vi "Taskbar Setup.vi"(4 "error in (no error)":errorcluster, 5 "DEV Icon Path (empty)":path, 6 "Tooltip Text (\"\")":string, 7 "Window Name (\"\")":string) -> (0 "error out":errorcluster, 1 "hIcon":i32, 2 "hWnd":T2, 3 "siwutil32":T1)   [LabVIEW 2011]
uses:
  SI.LIB/WIN32/WinUSER/Windows/hWnd.ctl
  SI.LIB/WIN32/SIWUTIL32/siwutil32.ctl
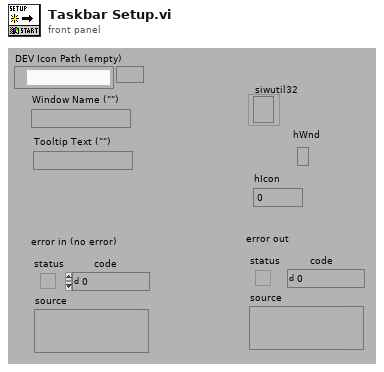
[diagram p1: front panel]
types:
  T1 = typedef "siwutil32.ctl" = refnum<k7>
  T2 = typedef "hWnd.ctl" = refnum<k1>
  T3 = enum32{"invalid app kind", "Development System", "Run Time System", "Student Edition", "Embedded LabVIEW", "Evaluation", "Custom"}
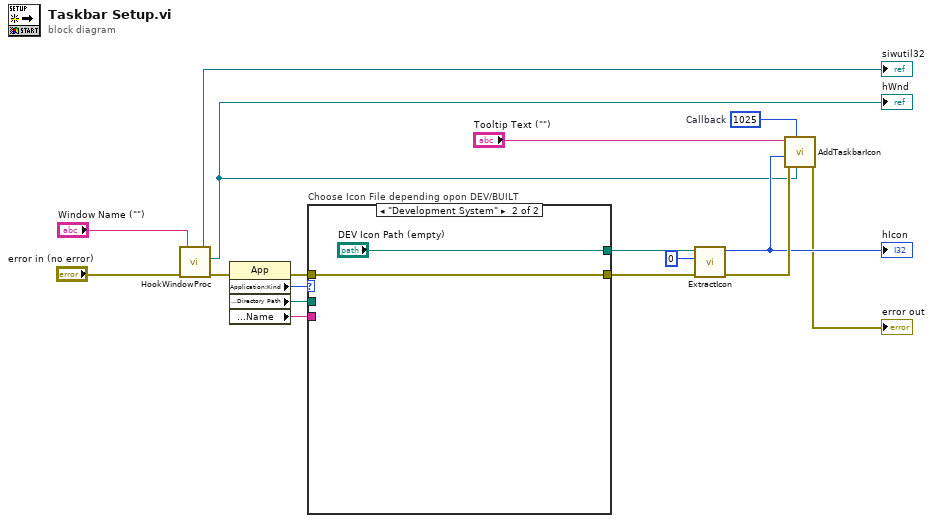
[diagram p0: block diagram]
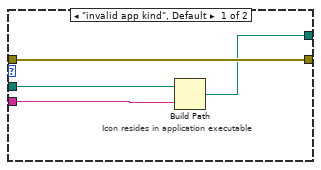
[diagram p2: hidden frame]
diagram:
  w15 = 1025  # Callback
  n1 = call "HookWindowProc.vi"("error in (no error)"="error in (no error)", "Window (\"\" - Parent)"="Window Name (\"\")") -> ("error out"=w9:errorcluster, "hWnd"=w11:T2, "siwutil32"=→"siwutil32":T1)  [unwired: 1 in, 2 out]
  "hWnd" <- w11
  n2 = property class="App"(error in=w9) -> (error out=w7:errorcluster, "Application:Kind"=w8:T3, "Application:Directory Path"=w6:path, "Application:Name"=w5:string)  [unwired: 1 in, 1 out]
  n3 = case "Choose Icon File depending opon DEV/BUILT" shown="\"Development System\"" w8 {
    tunnel: w7 -> [w19 w23]
    tunnel: w6 -> [w21 _]
    tunnel: w5 -> [w20 _]
    tunnel: [w19 w23] -> w4
    tunnel: [w18 "DEV Icon Path (empty)"] -> w3
    frame "invalid app kind", Default {
      # "Icon resides in application executable"
      n4 = Build Path(base path=w21, name or relative path=w20) -> (appended path=w18:path)
    }
    frame "Development System" {
    }
  }
  n5 = call "ExtractIcon.vi"("error in (no error)"=w4, "IconIndex (0)"=0 ("t"), "Path to Icon file (*.exe, *.dll, *.ico)"=w3) -> ("error out"=w17:errorcluster, "hIcon"=w16:i32)  [unwired: 3 out]
  "hIcon" <- w16
  n6 = call "AddTaskbarIcon.vi"("hWnd (NULL)"=w11, "Callback Message\n(0 - NULL)"=w15, "error in (no error)"=w17, "hIcon (NULL)"=w16, "Tooltip Text (\"\")"="Tooltip Text (\"\")") -> ("error out"=→"error out":errorcluster)  [unwired: 1 in, 5 out]
